vi "7495.vi"(4 "Clk 1\nR-Shift":bool, 5 "Serial\nInput":bool, 6 "Clk 2\nL-Shift":bool, 7 "Mode\nControl":bool, 8 "D":bool, 9 "C":bool, 10 "B":bool, 11 "A":bool) -> (0 "OD":bool, 1 "OC":bool, 2 "OB":bool, 3 "OA":bool)   [LabVIEW 2012]
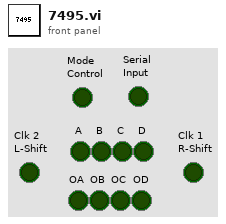
[diagram p1: front panel]
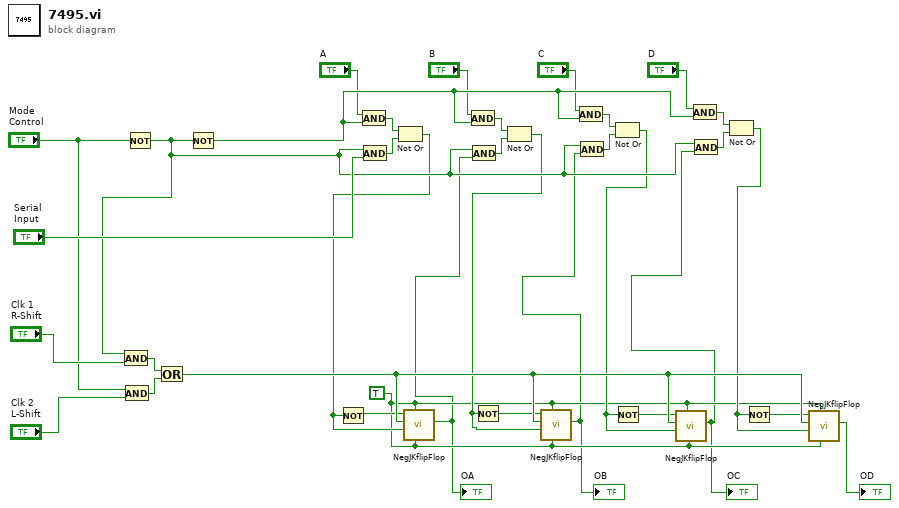
[diagram p0: block diagram]
diagram:
  w4 = TRUE
  n1 = And(x="Mode\nControl", y="Clk 2\nL-Shift") -> (x .and. y?=w26:bool)
  n2 = Not(x="Mode\nControl") -> (.not. x?=w15:bool)
  n3 = And(x=w15, y="Clk 1\nR-Shift") -> (x .and. y?=w25:bool)
  n4 = Or(x=w25, y=w26) -> (x .or. y?=w14:bool)
  n5 = Not(x=w15) -> (.not. x?=w22:bool)
  n6 = And(x="A", y=w22) -> (x .and. y?=w34:bool)
  n7 = And(x=w15, y="Serial\nInput") -> (x .and. y?=w33:bool)
  n8 = Not Or(1:w33, 2:w34) -> (0:w11:bool)
  n9 = Not(x=w11) -> (.not. x?=w12:bool)
  n10 = call "NegJKflipFlop.vi"("R"=w4, "S"=w4, "K"=w11, "Clk"=w14, "J"=w12) -> ("Q"=w3:bool)  [unwired: 5 in, 1 out]
  "OA" <- w3
  n11 = And(x="B", y=w22) -> (x .and. y?=w31:bool)
  n12 = And(x=w15, y=w3) -> (x .and. y?=w32:bool)
  n13 = Not Or(1:w32, 2:w31) -> (0:w9:bool)
  n14 = Not(x=w9) -> (.not. x?=w10:bool)
  n15 = call "NegJKflipFlop.vi"("R"=w4, "S"=w4, "K"=w9, "Clk"=w14, "J"=w10) -> ("Q"=w2:bool)  [unwired: 5 in, 1 out]
  "OB" <- w2
  n16 = And(x="C", y=w22) -> (x .and. y?=w30:bool)
  n17 = And(x=w15, y=w2) -> (x .and. y?=w29:bool)
  n18 = Not Or(1:w29, 2:w30) -> (0:w7:bool)
  n19 = Not(x=w7) -> (.not. x?=w8:bool)
  n20 = call "NegJKflipFlop.vi"("R"=w4, "S"=w4, "K"=w7, "Clk"=w14, "J"=w8) -> ("Q"=w1:bool)  [unwired: 5 in, 1 out]
  "OC" <- w1
  n21 = And(x="D", y=w22) -> (x .and. y?=w27:bool)
  n22 = And(x=w15, y=w1) -> (x .and. y?=w28:bool)
  n23 = Not Or(1:w28, 2:w27) -> (0:w5:bool)
  n24 = Not(x=w5) -> (.not. x?=w6:bool)
  n25 = call "NegJKflipFlop.vi"("R"=w4, "S"=w4, "K"=w5, "Clk"=w14, "J"=w6) -> ("Q"=→"OD":bool)  [unwired: 5 in, 1 out]
